vi "Generate Pulsed BPSK Filter Coefficients.vi"(8 "error in":errorcluster, 10 "samples per symbol":i32) -> (0 "error out":errorcluster, 1 "filter length (samples)":u16, 2 "pulse shaping filter coefficients":dbl[](array[numeric]), 3 "symmetric filter coefficients":T1)   [LabVIEW 2023, in "Pulsed BPSK Host Support.lvlib"]
uses:
  Pulsed BPSK Host Support.lvlib
  <vilib>/addons/Modulation/Analog/support/mod_Set Error Source.vi
  <vilib>/addons/Modulation/Digital/Support/Common/Validators/mod_Generate Filter Coefficients Validate.vi
  <vilib>/addons/Modulation/Digital/General/subVIs/mod_Generate Filter Coefficients.vi
  <vilib>/addons/Modulation/niDMT.lvlib
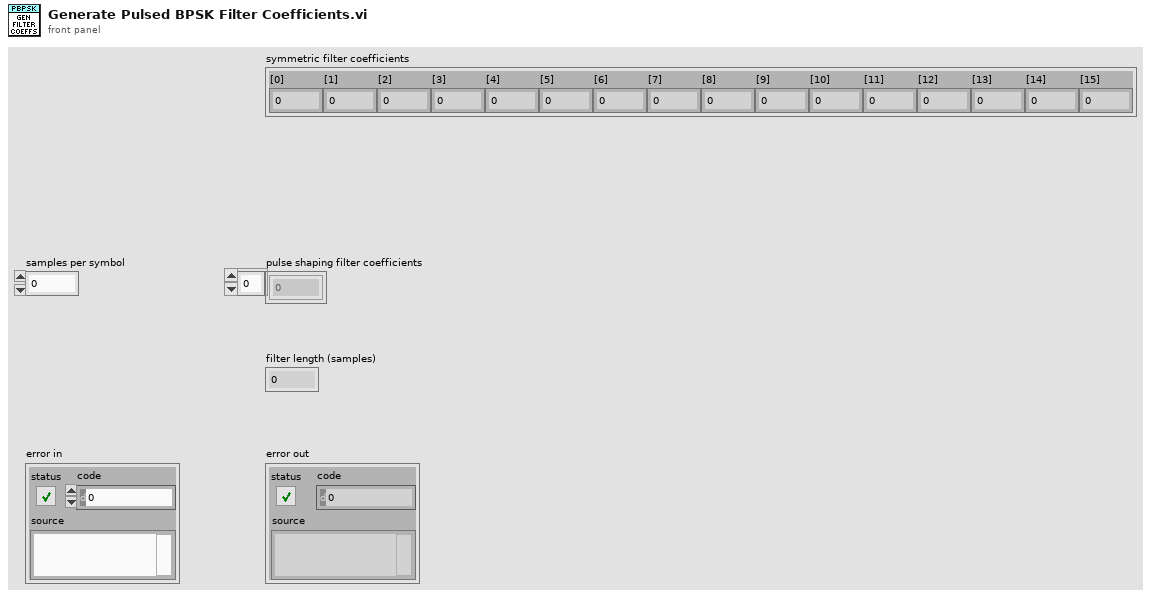
[diagram p1: front panel]
types:
  T1 = cluster{"[0]":fxp<+/-,16,1>, "[1]":fxp<+/-,16,1>, "[2]":fxp<+/-,16,1>, "[3]":fxp<+/-,16,1>, "[4]":fxp<+/-,16,1>, "[5]":fxp<+/-,16,1>, "[6]":fxp<+/-,16,1>, "[7]":fxp<+/-,16,1>, "[8]":fxp<+/-,16,1>, "[9]":fxp<+/-,16,1>, "[10]":fxp<+/-,16,1>, "[11]":fxp<+/-,16,1>, "[12]":fxp<+/-,16,1>, "[13]":fxp<+/-,16,1>, "[14]":fxp<+/-,16,1>, "[15]":fxp<+/-,16,1>}
  T2 = cluster{"TX Filter":enum16{"none", "Raised Cosine", "Root Raised Cos", "Gaussian"}, "Alpha":dbl, "Filter Length (symbols)":i32}
  T3 = enum16{"FSK", "PSK", "QAM", "MSK", "PAM", "ASK", "CPM"}
  T4 = enum16{"none", "Raised Cosine", "Root Raised Cos", "Gaussian"}
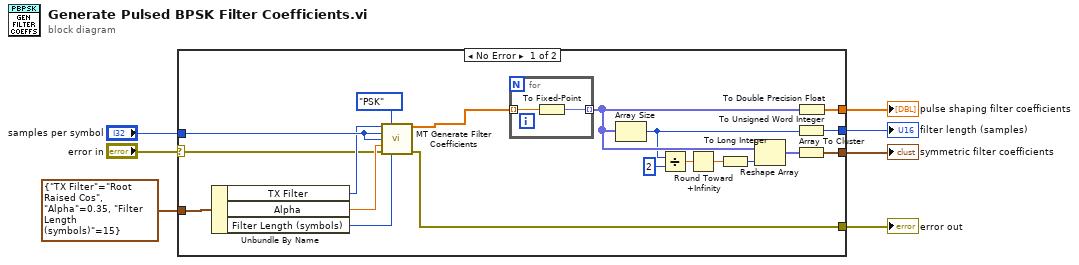
[diagram p0: block diagram]
diagram:
  n1 = case shown="No Error" "error in" {
    selector: "error in" -> [w16 w29]
    tunnel: "samples per symbol" -> [w26 _]
    tunnel: [w24 _] -> w6
    tunnel: [w23 _] -> w5
    tunnel: [w22 _] -> w4
    tunnel: T2 {"TX Filter"=enum."Root Raised Cos", "Alpha"=0.35, "Filter Length (symbols)"=15} ("Filter Parameters") -> [w18 _]
    tunnel: [w15 w29] -> w1
    frame No Error {
      n2 = Unbundle By Name(w18) -> ("TX Filter"=w19:T4, "Alpha"=w20:dbl, "Filter Length (symbols)"=w21:i32)
      n3 = call <vilib>:"MT Generate Filter Coefficients.vi"("pulse shaping filter (none)"=w19, "modulation type"=T3."PSK", "pulse shaping samples per symbol (16)"=w26, "matched samples per symbol (16)"=w26, "filter parameter"=w20, "error in (no error)"=w16, "filter length (symbols)"=w21) -> ("pulse shaping filter coefficients"=w8:dbl[], "error out"=w15:errorcluster)  [unwired: 6 in, 1 out]
      n4 = for {
        tunnel: w8 -> [w28] mode=indexing
        tunnel: [w27] -> w14 mode=indexing
        n5 = To Fixed-Point(number=w28) -> (fixed-point=w27:fxp<+/-,16,1>)  [unwired: 1 in]
      }
      n6 = Array Size(array=w14) -> (size(s)=w13:i32)
      n7 = Divide(x=w13, y=2) -> (x/y=w11:dbl)
      n8 = Round Toward +Infinity(x=w11) -> (ceil(x): smallest int >= x=w10:dbl)
      n9 = To Long Integer(number=w10) -> (32bit integer=w9:i32)
      n10 = Reshape Array(w14, w9) -> (w25:fxp<+/-,16,1>[])
      n11 = To Unsigned Word Integer(number=w13) -> (unsigned 16bit integer=w23:u16)
      n12 = Array To Cluster(array=w25) -> (cluster=w22:T1)
      n13 = To Double Precision Float(number=w14) -> (double precision float=w24:dbl[])
    }
    frame Error {
    }
  }
  "pulse shaping filter coefficients" <- w6
  "filter length (samples)" <- w5
  "symmetric filter coefficients" <- w4
  "error out" <- w1
